vi "Delay count.vi"(1 "Finished Late? [i-1]":bool) -> (0 "Count":u32)   [LabVIEW 2018]
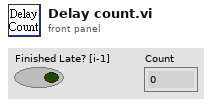
[diagram p1: front panel]
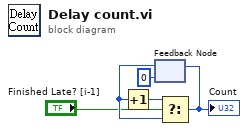
[diagram p0: block diagram]
diagram:
  n1 = feedback #1(u32 0) -> (w4:u32)
  n2 = Increment(x=w4) -> (x+1=w3:u32)
  n3 = Select(t=w3, s="Finished Late? [i-1]", f=w4) -> (s? t:f=w2:u32)
  "Count" <- w2
  n4 = feedback-in #1(w2) -> ()
